vi "Queue slowdown warning.vi"(9 "# elements in queue in":i32) -> ()   [LabVIEW 2017]
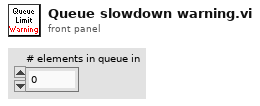
[diagram p1: front panel]
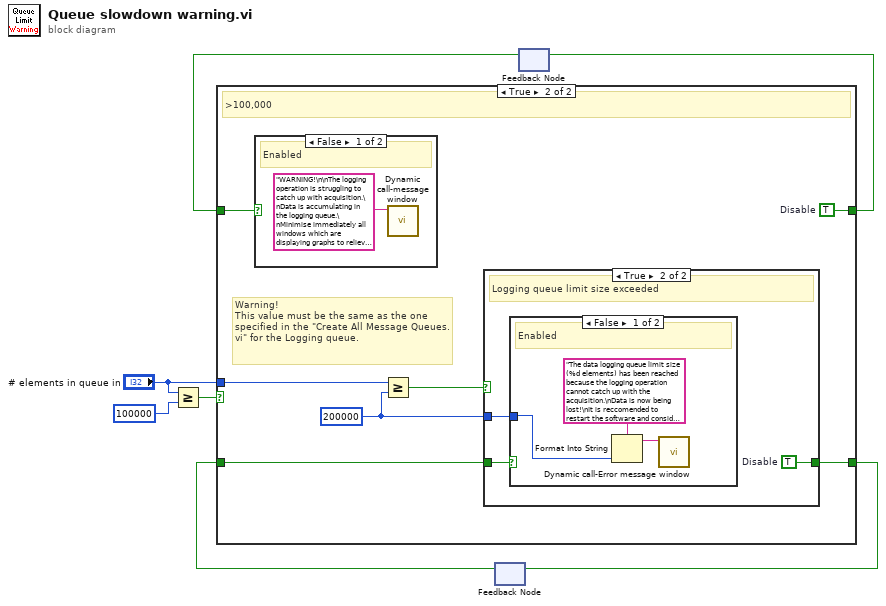
[diagram p0: block diagram]
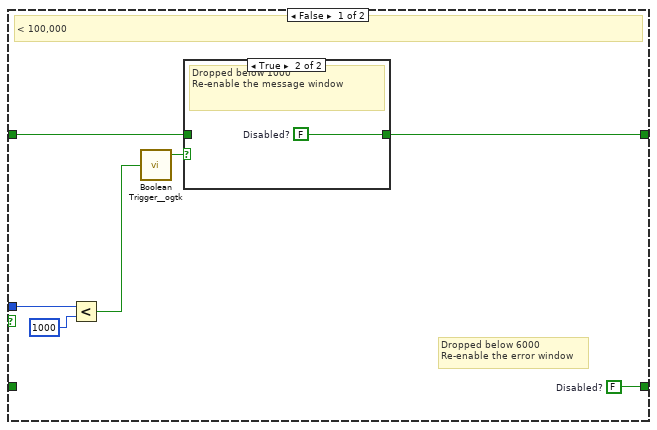
[diagram p2: hidden frame]
diagram:
  n1 = Greater Or Equal?(x="# elements in queue in", y=100000) -> (x >= y?=w3:bool)
  n2 = feedback #1() -> (w1:bool)  [unwired: 1 in]
  n3 = feedback #2() -> (w4:bool)  [unwired: 1 in]
  n4 = case shown="True" w3 {
    tunnel: "# elements in queue in" -> [w13 w23]
    tunnel: [w10 w21] -> w5
    tunnel: w4 -> [w9 w20]
    tunnel: [w8 w19] -> w2
    tunnel: w1 -> [_ w18]
    frame False {
      w8 = FALSE  # Disabled?
      # "Dropped below 6000\nRe-enable the error window"
      # "< 100,000"
      n5 = Less?(x=w13, y=1000) -> (x < y?=w12:bool)
      n6 = call <userlib>:"Boolean Trigger__ogtk.vi"("Boolean Input"=w12) -> ("Rising Edge"=w11:bool)  [unwired: 1 in, 1 out]
      n7 = case shown="True" w11 {
        tunnel: [w15 w16] -> w10
        tunnel: w9 -> [w15 _]
        frame False {
          # "Idle"
        }
        frame True {
          w16 = FALSE  # Disabled?
          # "Dropped below 1000\nRe-enable the message window"
        }
      }
    }
    frame True {
      w21 = TRUE  # Disable
      w17 = 200000 ("y")
      # "Warning!\nThis value must be the same as the one specified in the \"Create All Message Queues.vi\" for the Logging queue."
      # ">100,000"
      n8 = case shown="False" w20 {
        frame False {
          # "Enabled"
          n9 = call "Dynamic call-message window.vi"("Message"="WARNING!\n\nThe logging operation is struggling to catch up with acquisition.\nData is accumulating in the logging queue.\nMinimise immediately all windows which are displaying graphs to relieve the processor.\nConsider using a higher dwell time or a smaller frame size." ("Error Source")) -> ()  [unwired: 10 in, 1 out]
        }
        frame True {
          # "Disabled"
        }
      }
      n10 = Greater Or Equal?(x=w23, y=w17) -> (x >= y?=w22:bool)
      n11 = case shown="True" w22 {
        tunnel: [w25 w28] -> w19
        tunnel: w18 -> [w25 w27]
        tunnel: w17 -> [_ w26]
        frame False {
          # "<50000"
        }
        frame True {
          w28 = TRUE  # Disable
          # "Logging queue limit size exceeded"
          n12 = case shown="False" w27 {
            tunnel: w26 -> [w29 _]
            frame False {
              # "Enabled"
              n13 = Format Into String(format string="The data logging queue limit size (%d elements) has been reached because the logging operation cannot catch up with the acquisition.\nData is now being lost!\nIt is reccomended to restart the software and consider using a higher dwell time or a smaller frame size." ("Error Source"), w29) -> (resulting string=w30:string)  [unwired: 2 in, 1 out]
              n14 = call "Dynamic call-Error message window.vi"("Error Message"=w30) -> ()  [unwired: 10 in, 1 out]
            }
            frame True {
              # "Disabled"
            }
          }
        }
      }
    }
  }
  n15 = feedback-in #1(w2) -> ()
  n16 = feedback-in #2(w5) -> ()
